vi "Stream_DataSent.vi"(8 "error in (no error)":errorcluster, 9 "data":variant, 10 "streams":variant, 11 "Qbus":refnum<class "Qbus.lvclass">) -> (0 "error out":errorcluster, 2 "streams out":variant)   [LabVIEW 2017, in "FileManager.lvlib"]
uses:
  <vilib>/addons/InsightCM/Devices/Shared/Common/FileManager/FileManager.lvlib
  <vilib>/addons/Qbus/Qbus.lvclass
  <vilib>/addons/InsightCM/Devices/Shared/Common/FileManager/controls/StreamState.ctl
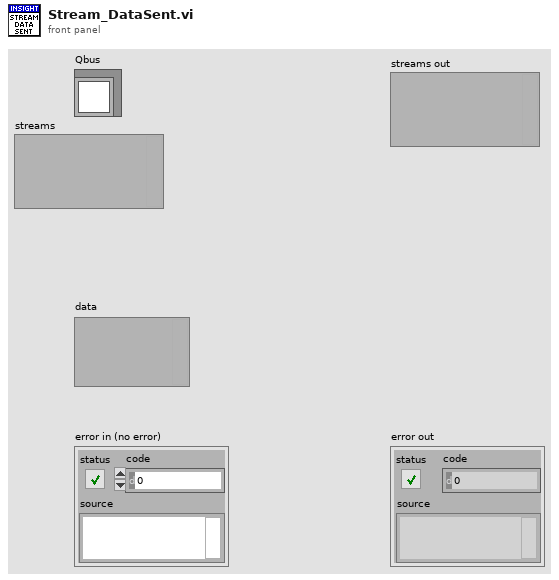
[diagram p1: front panel]
types:
  T1 = typedef "FileManager.lvlib/StreamState.ctl" = cluster{"DataGroup":string, "Stream Id":string, "LastBlock":bool, "TotalBlocks":i32, "BlocksSent":i32, "Device":string}
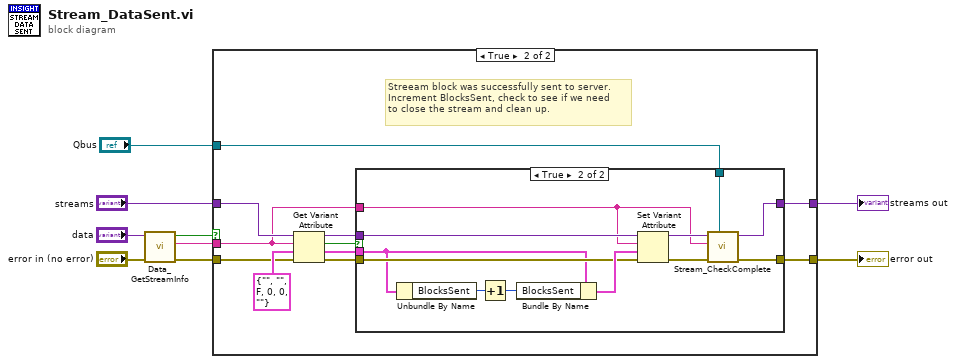
[diagram p0: block diagram]
diagram:
  n1 = call <vilib>:"Data_GetStreamInfo.vi"("error in (no error)"="error in (no error)", "data"="data") -> ("error out"=w7:errorcluster, "stream Id"=w6:string, "found"=w1:bool)  [unwired: 6 in, 1 out]
  n2 = case shown="True" w1 {
    tunnel: [w10 w16] -> w9
    tunnel: [w11 w14] -> w3
    tunnel: "streams" -> [w11 w18]
    tunnel: w7 -> [w10 w17]
    tunnel: w6 -> [_ w13]
    tunnel: "Qbus" -> [_ w15]
    frame False {
      # "Not a stream block."
    }
    frame True {
      # "Streeam block was successfully sent to server.\nIncrement BlocksSent, check to see if we need\nto close the stream and clean up."
      n3 = Get Variant Attribute(Variant=w18, name=w13, default value (empty Variant)=T1 {"DataGroup"="", "Stream Id"="", "LastBlock"=FALSE, "TotalBlocks"=0, "BlocksSent"=0, "Device"=""} ("Stream"), error in=w17) -> (duplicate Variant=w20:variant, found=w12:bool, value=w19:T1, error out=w21:errorcluster)
      n4 = case shown="True" w12 {
        tunnel: w21 -> [w23 w35]
        tunnel: w20 -> [w24 w34]
        tunnel: w19 -> [_ w33]
        tunnel: [w23 w29] -> w16
        tunnel: w15 -> [_ w28]
        tunnel: [w24 w26] -> w14
        tunnel: w13 -> [_ w25]
        frame False {
          # "If sending backlogged stream and that stream has already been finished,\n there won't be an entry for that stream in the 'streams' variant."
        }
        frame True {
          n5 = Unbundle By Name(w33) -> ("BlocksSent"=w32:i32)
          n6 = Increment(x=w32) -> (x+1=w31:i32)
          n7 = Bundle By Name(cluster=w33, "BlocksSent"=w31) -> (w36:T1)
          n8 = Set Variant Attribute(Variant=w34, name=w25, value=w36, error in=w35) -> (Variant out=w27:variant, error out=w30:errorcluster)  [unwired: 1 out]
          n9 = call <vilib>:"Stream_CheckComplete.vi"("Qbus in"=w28, "error in (no error)"=w30, "stream Id"=w25, "streams in"=w27) -> ("error out"=w29:errorcluster, "streams out"=w26:variant)  [unwired: 6 in]
        }
      }
    }
  }
  "error out" <- w9
  "streams out" <- w3
